vi "IVIDMM-Triggered-Readout.vi"() -> ()   [LabVIEW 2016, in "IVI_DMM.lvlib"]
uses:
  IVI_DMM.lvlib
panel:
  in  "sample trigger (Immediate)":i32(ring)=10 items=["Immediate"=1, "External"=2, "Software Trigger Function"=3, "Interval"=10, "PXI TRIG0 or VXI TTL0"=111, "PXI TRIG1 or VXI TTL1"=112, "PXI TRIG2 or VXI TTL2"=113, "PXI TRIG3 or VXI TTL3"=114, "PXI TRIG4 or VXI TTL4"=115, "PXI TRIG5 or VXI TTL5"=116, "PXI TRIG6 or VXI TTL6"=117, "PXI TRIG7 or VXI TTL7"=118, "ECL0"=119, "ECL1"=120, "PXI Star"=131, "RTSI 0"=140, "RTSI 1"=141, "RTSI 2"=142, "RTSI 3"=143, "RTSI 4"=144, "RTSI 5"=145, "RTSI 6"=146]
  in  "trigger source (Immediate)":i32(ring)=1 items=["Immediate"=1, "External"=2, "Software Trigger Function"=3, "PXI TRIG0 or VXI TTL0"=111, "PXI TRIG1 or VXI TTL1"=112, "PXI TRIG2 or VXI TTL2"=113, "PXI TRIG3 or VXI TTL3"=114, "PXI TRIG4 or VXI TTL4"=115, "PXI TRIG5 or VXI TTL5"=116, "PXI TRIG6 or VXI TTL6"=117, "PXI TRIG7 or VXI TTL7"=118, "ECL0"=119, "ECL1"=120, "PXI Star"=131, "RTSI 0"=140, "RTSI 1"=141, "RTSI 2"=142, "RTSI 3"=143, "RTSI 4"=144, "RTSI 5"=145, "RTSI 6"=146]
  in  "Slave (F)":bool
  in  "IVI Logical Name":refnum<k15>
  out "dt":dbl[unit] format="%.3f"
  out "Nof points":i32 caption="actual number of points"
  out "Aperture":dbl[unit]
  out "Graph":dbl[](graph)
  in  "sample count":i32=10 caption="sample count (1)"
  in  "sample interval":dbl[unit]=0.02 caption="sample interval (0.0 s)" format="%.3f"
  out "error out":errorcluster
  in  "Stop":bool
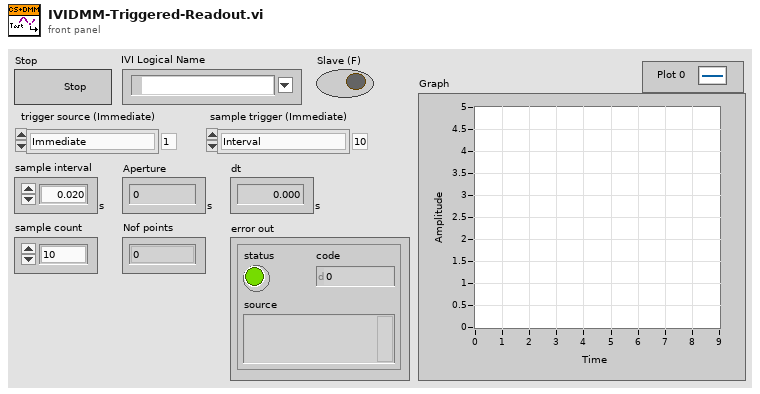
[diagram p1: front panel]
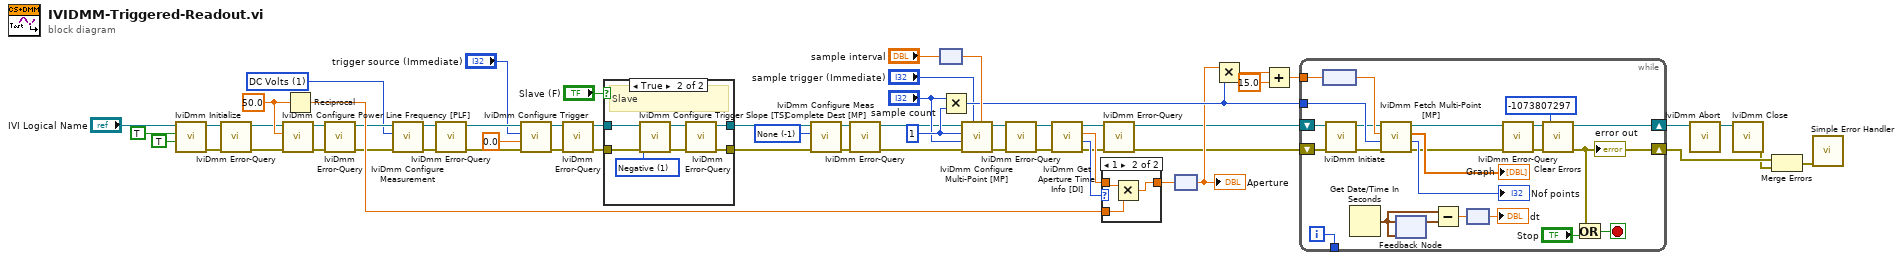
[diagram p0: block diagram]
diagram:
  w48 = -1 items=["None"=-1, "External"=2, "PXI TRIG0 or VXI TTL0"=111, "PXI TRIG1 or VXI TTL1"=112, "PXI TRIG2 or VXI TTL2"=113, "PXI TRIG3 or VXI TTL3"=114, "PXI TRIG4 or VXI TTL4"=115, "PXI TRIG5 or VXI TTL5"=116, "PXI TRIG6 or VXI TTL6"=117, "PXI TRIG7 or VXI TTL7"=118, "ECL0"=119, "ECL1"=120, "PXI Star"=131, "RTSI 0"=140, "RTSI 1"=141, "RTSI 2"=142, "RTSI 3"=143, "RTSI 4"=144, "RTSI 5"=145, "RTSI 6"=146] ("meas complete dest (None)")
  w33 = 1 ("trigger count (1)")
  w3 = 1 items=["DC Volts"=1, "AC Volts"=2, "DC Current"=3, "AC Current"=4, "2 Wire Resistance"=5, "4 Wire Resistance"=101, "AC + DC Volts"=106, "AC + DC Current"=107, "Frequency"=104, "Period"=105, "Temperature"=108] ("measurement function (DC Volts)")
  w44 = 50.0 ("power line frequency (60.0 Hz)")
  n1 = call <vilib>:"IviDmm Initialize.vi"("reset device (True)"=TRUE ("Reset (F)"), "id query (True)"=TRUE, "logical name (\"SampleDmm\")"="IVI Logical Name") -> ("error out"=w28:errorcluster, "instrument handle out"=w31:refnum<k15>)  [unwired: 7 in]
  n2 = call <vilib>:"IviDmm Error-Query.vi"("error in (no error)"=w28, "instrument handle"=w31) -> ("error out"=w27:errorcluster, "instrument handle out"=w29:refnum<k15>)  [unwired: 6 in, 2 out]
  n3 = call <vilib>:"IviDmm Configure Power Line Frequency [PLF].vi"("error in (no error)"=w27, "power line frequency (60.0 Hz)"=w44, "instrument handle"=w29) -> ("error out"=w25:errorcluster, "instrument handle out"=w49:refnum<k15>)  [unwired: 7 in]
  n4 = Reciprocal(x=w44) -> (1/x=w43:dbl)
  n5 = call <vilib>:"IviDmm Error-Query.vi"("error in (no error)"=w25, "instrument handle"=w49) -> ("error out"=w24:errorcluster, "instrument handle out"=w26:refnum<k15>)  [unwired: 6 in, 2 out]
  n6 = call <vilib>:"IviDmm Configure Measurement.vi"("error in (no error)"=w24, "measurement function (DC Volts)"=w3, "instrument handle"=w26) -> ("error out"=w22:errorcluster, "instrument handle out"=w38:refnum<k15>)  [unwired: 7 in]
  n7 = call <vilib>:"IviDmm Error-Query.vi"("error in (no error)"=w22, "instrument handle"=w38) -> ("error out"=w21:errorcluster, "instrument handle out"=w23:refnum<k15>)  [unwired: 6 in, 2 out]
  n8 = call <vilib>:"IviDmm Configure Trigger.vi"("error in (no error)"=w21, "trigger delay (0.0 s)"=0.0, "trigger source (Immediate)"="trigger source (Immediate)", "instrument handle"=w23) -> ("error out"=w19:errorcluster, "instrument handle out"=w40:refnum<k15>)  [unwired: 6 in]
  n9 = call <vilib>:"IviDmm Error-Query.vi"("error in (no error)"=w19, "instrument handle"=w40) -> ("error out"=w18:errorcluster, "instrument handle out"=w20:refnum<k15>)  [unwired: 6 in, 2 out]
  n10 = case shown="True" "Slave (F)" {
    tunnel: w20 -> [w60 w67]
    tunnel: [w60 w63] -> w42
    tunnel: w18 -> [w59 w65]
    tunnel: [w59 w61] -> w41
    frame False {
      # "Master"
    }
    frame True {
      w64 = 1 items=["Positive", "Negative"] ("trigger slope (0: Positive)")
      # "Slave"
      n11 = call <vilib>:"IviDmm Configure Trigger Slope [TS].vi"("error in (no error)"=w65, "trigger slope (0: Positive)"=w64, "instrument handle"=w67) -> ("error out"=w62:errorcluster, "instrument handle out"=w66:refnum<k15>)  [unwired: 7 in]
      n12 = call <vilib>:"IviDmm Error-Query.vi"("error in (no error)"=w62, "instrument handle"=w66) -> ("error out"=w61:errorcluster, "instrument handle out"=w63:refnum<k15>)  [unwired: 6 in, 2 out]
    }
  }
  n13 = call <vilib>:"IviDmm Configure Meas Complete Dest [MP].vi"("error in (no error)"=w41, "meas complete dest (None)"=w48, "instrument handle"=w42) -> ("error out"=w16:errorcluster, "instrument handle out"=w37:refnum<k15>)  [unwired: 7 in]
  n14 = call <vilib>:"IviDmm Error-Query.vi"("error in (no error)"=w16, "instrument handle"=w37) -> ("error out"=w15:errorcluster, "instrument handle out"=w17:refnum<k15>)  [unwired: 6 in, 2 out]
  n15 = node("sample interval") -> (w35:dbl)
  n16 = Multiply(x="sample count", y=w33) -> (x*y=w34:i32)
  n17 = call <vilib>:"IviDmm Configure Multi-Point [MP].vi"("sample interval (0.0 s)"=w35, "sample trigger (Immediate)"="sample trigger (Immediate)", "error in (no error)"=w15, "sample count (1)"="sample count", "trigger count (1)"=w33, "instrument handle"=w17) -> ("error out"=w13:errorcluster, "instrument handle out"=w36:refnum<k15>)  [unwired: 4 in]
  n18 = call <vilib>:"IviDmm Error-Query.vi"("error in (no error)"=w13, "instrument handle"=w36) -> ("error out"=w12:errorcluster, "instrument handle out"=w14:refnum<k15>)  [unwired: 6 in, 2 out]
  n19 = call <vilib>:"IviDmm Get Aperture Time Info [DI].vi"("error in (no error)"=w12, "instrument handle"=w14) -> ("error out"=w11:errorcluster, "aperture time units"=w47:i32, "aperture time (sec)"=w46:dbl, "instrument handle out"=w58:refnum<k15>)  [unwired: 6 in]
  n20 = case shown="1" w47 {
    tunnel: w46 -> [w68 w71]
    tunnel: [w68 w69] -> w45
    tunnel: w43 -> [_ w70]
    frame 0, Default {
    }
    frame 1 {
      n21 = Multiply(x=w71, y=w70) -> (x*y=w69:dbl)
    }
  }
  n22 = call <vilib>:"IviDmm Error-Query.vi"("error in (no error)"=w11, "instrument handle"=w58) -> ("error out"=w6:errorcluster, "instrument handle out"=w7:refnum<k15>)  [unwired: 6 in, 2 out]
  n23 = node(w45) -> (w8:dbl[unit])
  "Aperture" <- w8
  n24 = Multiply(x=w8, y=w34) -> (x*y=w53:dbl[unit])
  n25 = Add(x=w53, y=dbl[unit] 15.0 ("x")) -> (x+y=w51:dbl[unit])
  n26 = while {
    shift-right: [w80] -> w56
    shift-left: w6 -> [w73]
    shift-right: [w82] -> w57
    shift-left: w7 -> [w75]
    tunnel: w51 -> [w83]
    tunnel: w34 -> [w92]
    tunnel: [w76] -> _
    i -> [w76]
    stop <- w91 stop-if-true
    n27 = node(w83) -> (w84:dbl)
    n28 = call <vilib>:"IviDmm Initiate.vi"("error in (no error)"=w73, "instrument handle"=w75) -> ("error out"=w72:errorcluster, "instrument handle out"=w74:refnum<k15>)  [unwired: 8 in]
    n29 = Get Date/Time In Seconds() -> (seconds since 1Jan1904=w88:timestamp)
    n30 = call <vilib>:"IviDmm Fetch Multi-Point [MP].vi"("error in (no error)"=w72, "array size (1)"=w92, "maximum time (5000 ms)"=w84, "instrument handle"=w74) -> ("error out"=w77:errorcluster, "actual number of points"=→"Nof points":i32, "reading array"=→"Graph":dbl[], "instrument handle out"=w78:refnum<k15>)  [unwired: 4 in]
    n31 = feedback #1(w88) -> (w87:timestamp)
    n32 = feedback-in #1(w88) -> ()
    n33 = Subtract(x=w88, y=w87) -> (x-y=w86:dbl)
    n34 = node(w86) -> (→"dt":dbl[unit])
    n35 = call <vilib>:"IviDmm Error-Query.vi"("error in (no error)"=w77, "instrument handle"=w78) -> ("error out"=w81:errorcluster, "instrument handle out"=w82:refnum<k15>)  [unwired: 6 in, 2 out]
    n36 = call <vilib>:"Clear Errors.vi"("error in (no error)"=w81, "specific error code to clear (0: all)"=-1073807297) -> ("error out"=w80:errorcluster)  [unwired: 4 in, 1 out]
    "error out" <- w80
    n37 = Or(x=w80, y="Stop") -> (x .or. y?=w91:bool)
  }
  n38 = call <vilib>:"IviDmm Abort.vi"("instrument handle"=w57) -> ("instrument handle out"=w10:refnum<k15>)  [unwired: 9 in, 1 out]
  n39 = call <vilib>:"IviDmm Close.vi"("instrument handle"=w10) -> ("error out"=w55:errorcluster)  [unwired: 10 in]
  n40 = Merge Errors(w56, w55) -> (w54:errorcluster)
  n41 = call <vilib>:"Simple Error Handler.vi"("error in (no error)"=w54) -> ()  [unwired: 4 in, 5 out]
